vi "Falling Edge.vi"(5 "Input":bool) -> (2 "Output":bool)   [LabVIEW 2012]
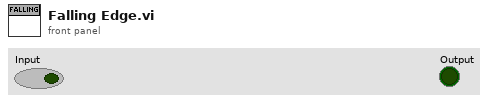
[diagram p1: front panel]
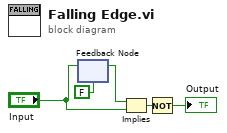
[diagram p0: block diagram]
diagram:
  n1 = feedback #1(FALSE ("Button 2")) -> (w1:bool)
  n2 = feedback-in #1("Input") -> ()
  n3 = Implies(1:"Input", 2:w1) -> (0:w4:bool)
  n4 = Not(x=w4) -> (.not. x?=→"Output":bool)
